vi "KE622x -- Set Standard Event Enable Reg State.vi"(0 "VISA Resource In":refnum<visa-resource-name>, 1 "Error Query (T)?":bool=TRUE, 7 "KE622x Standard Event Enable Reg":T1, 11 "error in (no error)":errorcluster) -> (4 "VISA Resource Out (dupl)":refnum<visa-resource-name>, 15 "error out":errorcluster)   [LabVIEW 2019, in "Keithley 622x.lvlib"]
doc: "Returns the bits in the 'Standard Event Enable' register of the Status Model. Note that only the used (named) bits are settable -- all other bits default to zero."
uses:
  Keithley 622x.lvlib
  Typedefs/KE622x -- Standard Event Enable Reg State.ctl
panel:
  out "Reg Num (dec)":u16 format="%0d"
  out "Reg Num (binary)":u16 format="%016b"
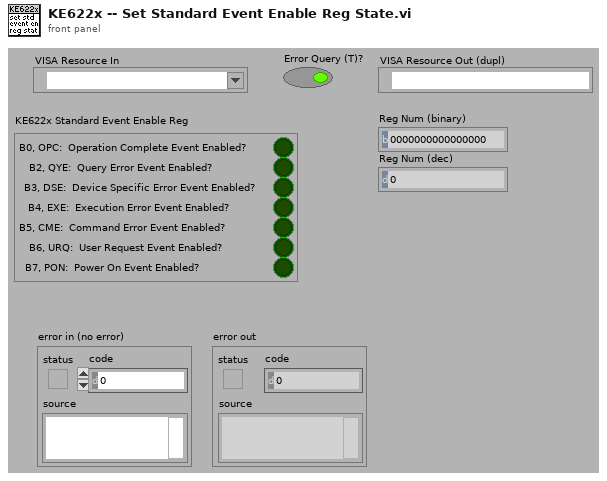
[diagram p1: front panel]
types:
  T1 = typedef "Keithley 622x.lvlib/KE622x -- Standard Event Enable Reg State.ctl" = cluster{"B0, OPC:  Operation Complete Event Enabled?":bool, "B2, QYE:  Query Error Event Enabled?":bool, "B3, DSE:  Device Specific Error Event Enabled?":bool, "B4, EXE:  Execution Error Event Enabled?":bool, "B5, CME:  Command Error Event Enabled?":bool, "B6, URQ:  User Request Event Enabled?":bool, "B7, PON:  Power On Event Enabled?":bool}
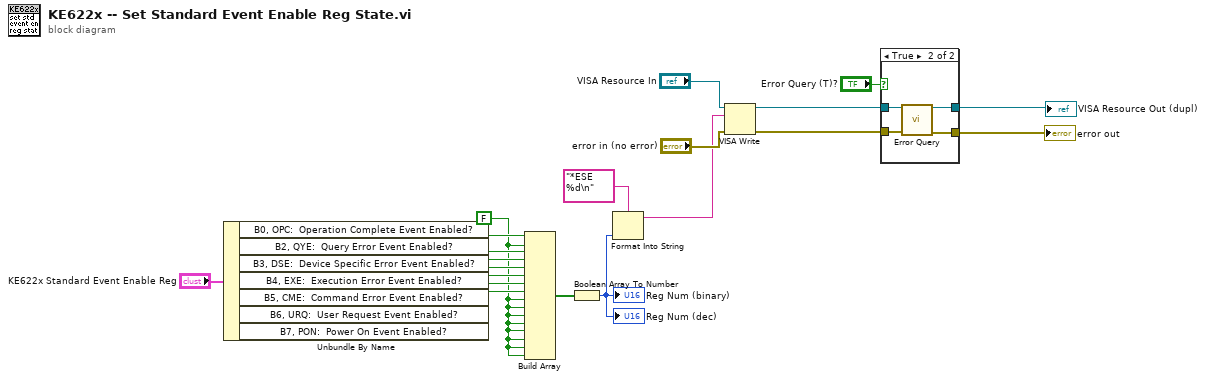
[diagram p0: block diagram]
diagram:
  w7 = FALSE
  n1 = Unbundle By Name("KE622x Standard Event Enable Reg") -> ("B0, OPC:  Operation Complete Event Enabled?"=w14:bool, "B2, QYE:  Query Error Event Enabled?"=w13:bool, "B3, DSE:  Device Specific Error Event Enabled?"=w12:bool, "B4, EXE:  Execution Error Event Enabled?"=w11:bool, "B5, CME:  Command Error Event Enabled?"=w10:bool, "B6, URQ:  User Request Event Enabled?"=w9:bool, "B7, PON:  Power On Event Enabled?"=w8:bool)
  n2 = Build Array(w14, w7, w13, w12, w11, w10, w9, w8, w7, w7, w7, w7, w7, w7, w7, w7) -> (w20:bool[])
  n3 = Boolean Array To Number(Boolean array=w20) -> (number=w17:u32)
  "Reg Num (binary)" <- w17
  "Reg Num (dec)" <- w17
  n4 = Format Into String(format string="*ESE %d\n" ("write buffer"), w17) -> (resulting string=w15:string)  [unwired: 2 in, 1 out]
  n5 = VISA Write(VISA resource name="VISA Resource In", write buffer=w15, error in (no error)="error in (no error)") -> (VISA resource name out=w3:refnum<visa-resource-name>, error out=w4:errorcluster)  [unwired: 1 out]
  n6 = case shown="True" "Error Query (T)?" {
    tunnel: w4 -> [w21 w26]
    tunnel: w3 -> [w22 w25]
    tunnel: [w21 w24] -> w1
    tunnel: [w22 w23] -> w2
    frame False {
    }
    frame True {
      n7 = call "Error Query.vi"("VISA Resource In"=w25, "error in (no error)"=w26) -> ("VISA Resource Out (dupl)"=w23:refnum<visa-resource-name>, "error out"=w24:errorcluster)  [unwired: 10 in, 2 out]
    }
  }
  "VISA Resource Out (dupl)" <- w2
  "error out" <- w1
